vi "Write FftView.vi"(8 "error in (no error)":errorcluster, 10 "FftView":T1, 11 "FFT in":refnum<class "FFT.lvclass">) -> (0 "error out":errorcluster, 3 "FFT out":refnum<class "FFT.lvclass">)   [LabVIEW 2014, in "AnalysisPlugins.lvlib" / "FFT.lvclass"]
uses:
  FFT.lvclass
  Typedefs/FftView.ctl
  FFT.lvclass/FFT.ctl
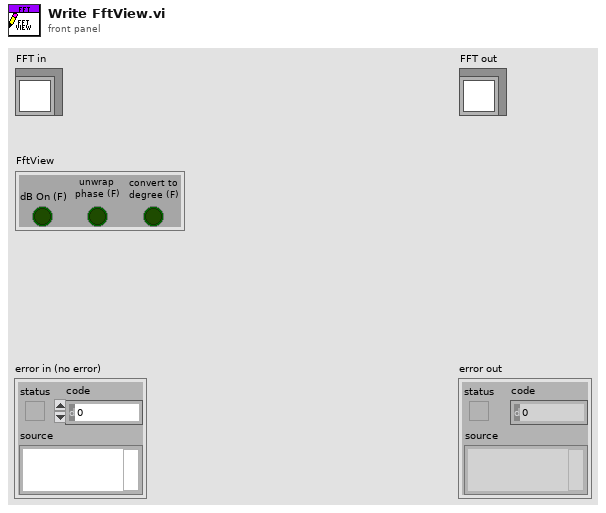
[diagram p1: front panel]
types:
  T1 = typedef "AnalysisPlugins.lvlib/FFT.lvclass/FftView.ctl" = cluster{"dB On (F)":bool, "unwrap phase (F)":bool, "convert to degree (F)":bool}
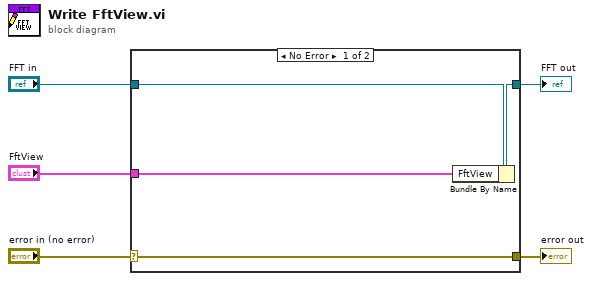
[diagram p0: block diagram]
diagram:
  n1 = case shown="No Error" "error in (no error)" {
    selector: "error in (no error)" -> [w9 w10]
    tunnel: [w9 w10] -> w4
    tunnel: [w7 w11] -> w2
    tunnel: "FFT in" -> [w8 w11]
    tunnel: "FftView" -> [w6 _]
    frame No Error {
      n2 = Bundle By Name(cluster=w8, "FftView"=w6) -> (w7:refnum<class "FFT.lvclass">)
    }
    frame Error {
    }
  }
  "error out" <- w4
  "FFT out" <- w2
